vi "FABR-Advance Sequence.vi"(0 "Runtime in":T2, 5 "Tickets in":T1[](array[typedef]), 7 "SCL in":T3[](array[typedef]), 11 "error in (no error)":errorcluster) -> (4 "Runtime thru":T2, 6 "Tickets thru":T1[](array[typedef]), 8 "SCL out":T3[](array[typedef]), 10 "finished":bool, 15 "error out":errorcluster)   [LabVIEW 2020]
uses:
  Typedefs/FABR-Stimulus Condition.ctl
  Typedefs/FABR-Runtime Data.ctl
  Typedefs/FABR-Stimulus Ticket.ctl
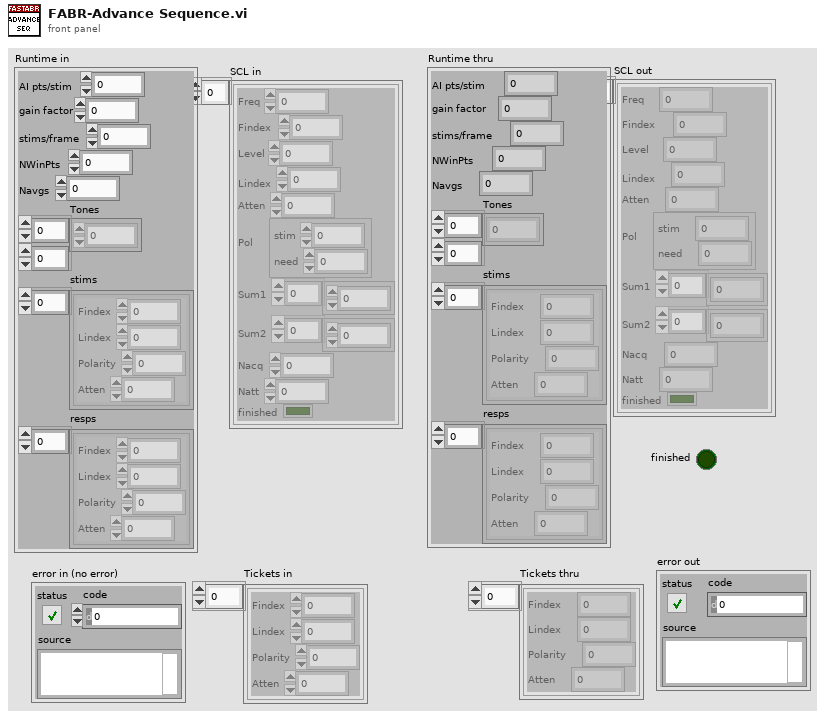
[diagram p1: front panel]
types:
  T1 = typedef "FABR-Stimulus Ticket.ctl" = cluster{"Findex":i32, "Lindex":i32, "Polarity":i32, "Atten":dbl}
  T2 = typedef "FABR-Runtime Data.ctl" = cluster{"AI pts/stim":i32, "gain factor":dbl, "stims/frame":i32, "NWinPts":i32, "Navgs":i32, "Tones":dbl[][], "stims":T1[], "resps":T1[]}
  T3 = typedef "FABR-Stimulus Condition.ctl" = cluster{"Freq":dbl, "Findex":i32, "Level":dbl, "Lindex":i32, "Atten":dbl, "Pol":cluster{"stim":i32, "need":i32}, "Sum1":dbl[], "Sum2":dbl[], "Nacq":i32, "Natt":i32, "finished":bool}
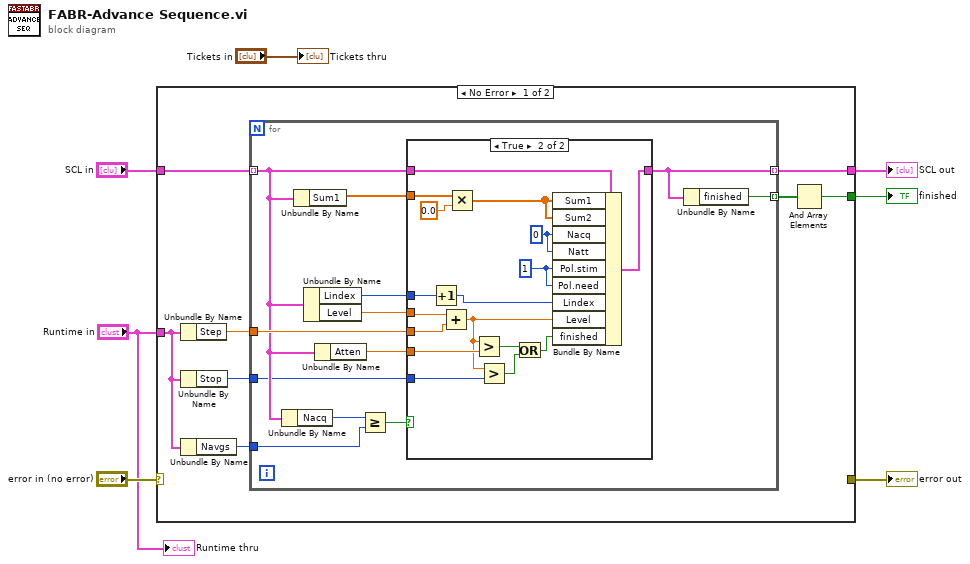
[diagram p0: block diagram]
diagram:
  n1 = case shown="No Error" "error in (no error)" {
    selector: "error in (no error)" -> [_ w47]
    tunnel: "Runtime in" -> [w12 _]
    tunnel: "SCL in" -> [w15 w46]
    tunnel: [_ w47] -> w5
    tunnel: [w10 w46] -> w3
    tunnel: [w8 _] -> w2
    frame No Error {
      n2 = Unbundle By Name(w12) -> ("Step"=w13:dbl)
      n3 = Unbundle By Name(w12) -> ("Stop"=w11:i32)
      n4 = Unbundle By Name(w12) -> ("Navgs"=w14:i32)
      n5 = for {
        tunnel: w15 -> [w20] mode=indexing
        tunnel: w14 -> [w27]
        tunnel: w13 -> [w21]
        tunnel: w11 -> [w18]
        tunnel: [w17] -> w10 mode=indexing
        tunnel: [w16] -> w9 mode=indexing
        n6 = Unbundle By Name(w20) -> ("Nacq"=w24:i32)
        n7 = Unbundle By Name(w20) -> ("Sum1"=w25:dbl[])
        n8 = Unbundle By Name(w20) -> ("Lindex"=w23:i32, "Level"=w22:dbl)
        n9 = Unbundle By Name(w20) -> ("Atten"=w19:dbl)
        n10 = Greater Or Equal?(x=w24, y=w27) -> (x >= y?=w26:bool)
        n11 = case shown="True" w26 {
          tunnel: w20 -> [w28 w45]
          tunnel: w25 -> [_ w44]
          tunnel: w23 -> [_ w40]
          tunnel: w22 -> [_ w38]
          tunnel: w21 -> [_ w37]
          tunnel: w19 -> [_ w36]
          tunnel: w18 -> [_ w33]
          tunnel: [w28 w30] -> w17
          frame False {
          }
          frame True {
            w29 = 1 ("Pol")
            w41 = 0 ("Nacq")
            n12 = Increment(x=w40) -> (x+1=w39:i32)
            n13 = Add(x=w38, y=w37) -> (x+y=w34:dbl)
            n14 = Multiply(x=w44, y=0.0) -> (x*y=w42:dbl[])
            n15 = Greater?(x=w34, y=w36) -> (0:w35:bool)
            n16 = Greater?(x=w34, y=w33) -> (0:w31:bool)
            n17 = Or(x=w35, y=w31) -> (x .or. y?=w32:bool)
            n18 = Bundle By Name(cluster=w45, "Sum1"=w42, "Sum2"=w42, "Nacq"=w41, "Natt"=w41, "Pol.stim"=w29, "Pol.need"=w29, "Lindex"=w39, "Level"=w34, "finished"=w32) -> (w30:T3)
          }
        }
        n19 = Unbundle By Name(w17) -> ("finished"=w16:bool)
      }
      n20 = And Array Elements(Boolean array=w9) -> (logical AND=w8:bool)
    }
    frame Error {
    }
  }
  "finished" <- w2
  "error out" <- w5
  "SCL out" <- w3
  "Runtime thru" <- "Runtime in"
  "Tickets thru" <- "Tickets in"
